vi "HiPace1200_Main.vi"() -> ()   [LabVIEW 2019]
panel:
  in  "audio_onoff":bool=TRUE caption="Audio\nAlarm"
  in  "control_onoff":bool=TRUE caption="Control"
  out "ack_ok":bool=TRUE
  out "motor_onoff":bool
  out "pump_st_onoff":bool
  out "temp_rotor":i16 caption="Rotor"
  out "temp_motor":i16 caption="Motor"
  out "temp_bearng":i16 caption="Bearing"
  out "temp_pmp_bot":i16 caption="Pump Bottom"
  out "temp_elec":i16 caption="Electric"
  out "temp_pwr_stg":i16 caption="Power Stage"
  out "gas_flow":i16 caption="sccm"
  out "accel":i16 caption="Accel."
  out "rot_speed_nom":i16 caption="Nominal"
  out "rot_speed_sp":i16 caption="Set Point"
  out "rot_speed_r":i16 caption="Reading"
  out "error_code":string caption="Error Code"
  in  "reconnect":bool
  in  "ack_error":bool
  in  "turn_off_motor":bool
  in  "turn_on_motor":bool
  in  "turn_off_pump_st":bool
  in  "turn_on_pump_st":bool
  in  "device_addr":u16=1 caption="Device addr."
  in  "port":u16=4196 caption="Port"
  in  "ip_addr":string="192.168.24.133" caption="IP addr."
  out "time":timestamp caption="Time" format="%<%Y-%m-%d %H:%M:%S>T"
  out "status":bool caption="Comm. status"
  in  "interval":u32=5000 caption="Interval"
  in  "stop":bool
  # "HiPace 1200:  Secondary IVC Pump"
  # "Pump Station"
  # "Rotation Speed"
  # "Hz"
  # "Hz"
  # "Hz"
  # "rpm/s"
  # "Temperature"
  # "Turbo Motor"
  # "degC"
  # "degC"
  # "degC"
  # "degC"
  # "degC"
  # "Error Code"
  # "degC"
  # "Gas Flow"
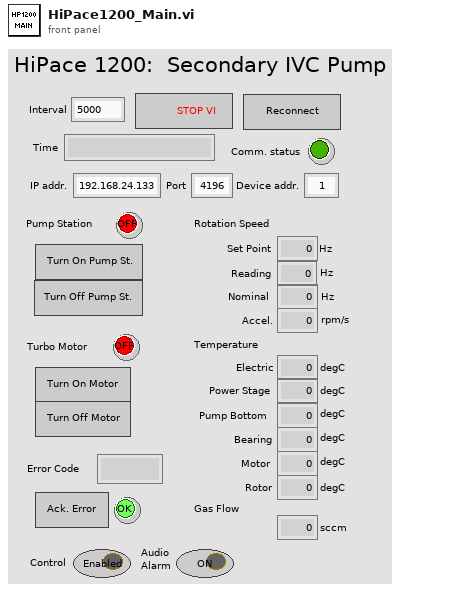
[diagram p1: front panel]
types:
  T1 = enum8{"Enabled", "Disabled", "Disabled and Grayed Out"}
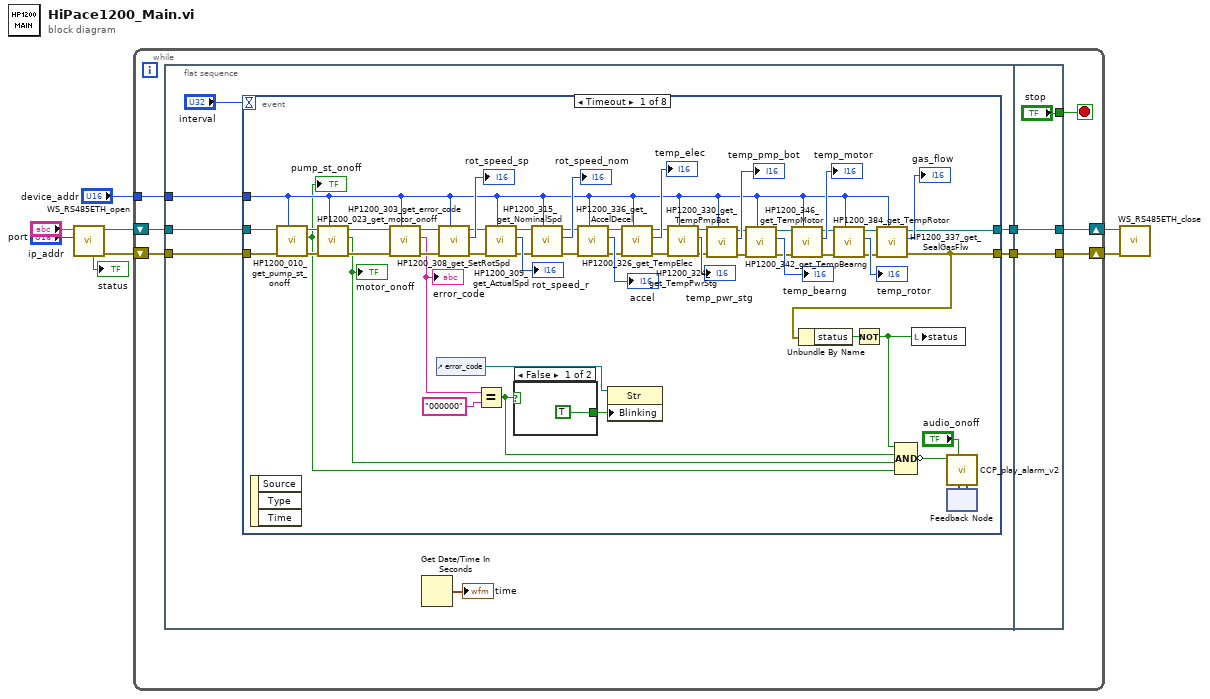
[diagram p0: block diagram]
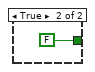
[diagram p2: hidden frame]
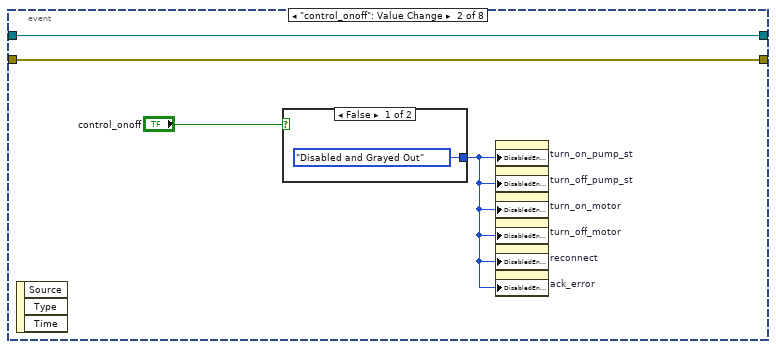
[diagram p3: hidden frame]
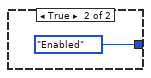
[diagram p4: hidden frame]
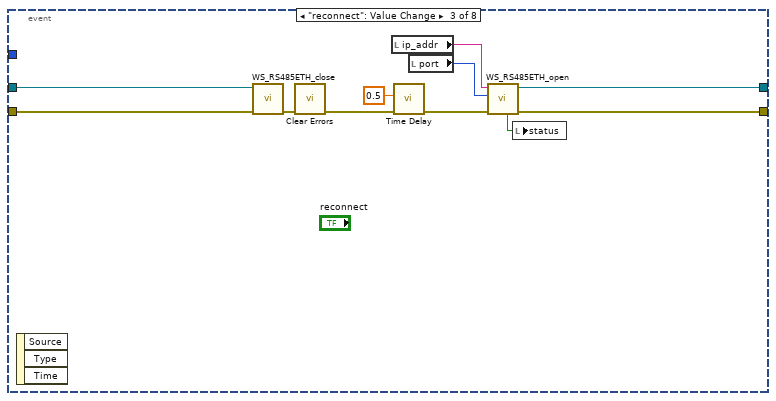
[diagram p5: hidden frame]
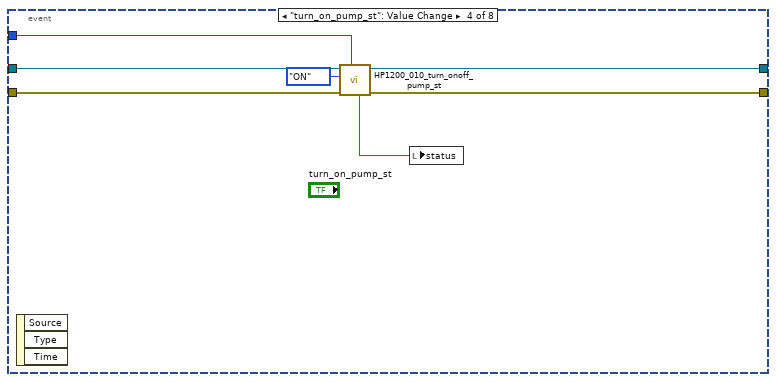
[diagram p6: hidden frame]
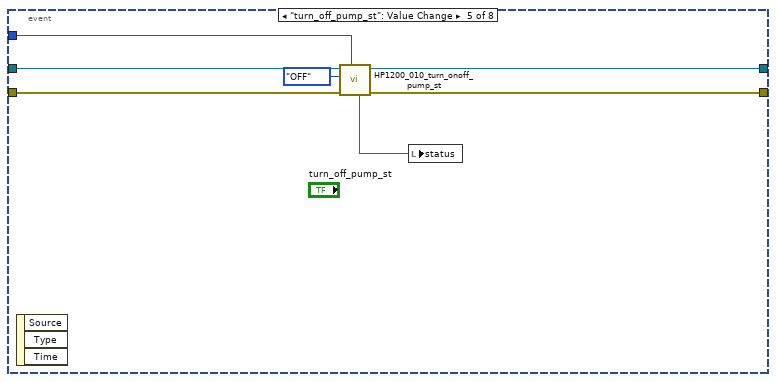
[diagram p7: hidden frame]
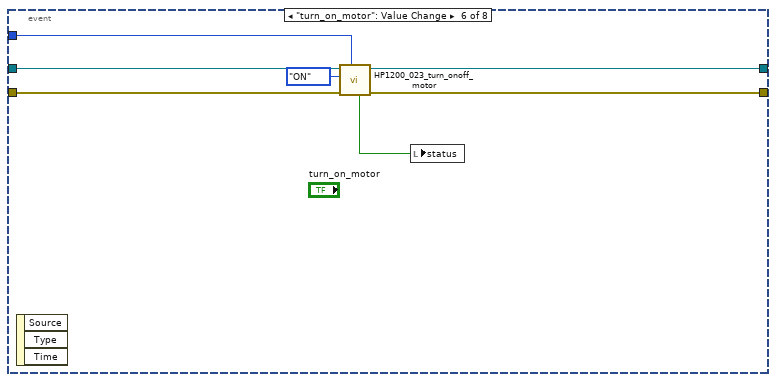
[diagram p8: hidden frame]
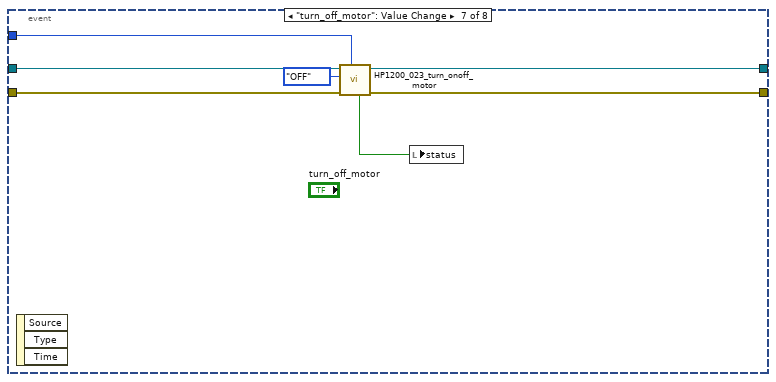
[diagram p9: hidden frame]
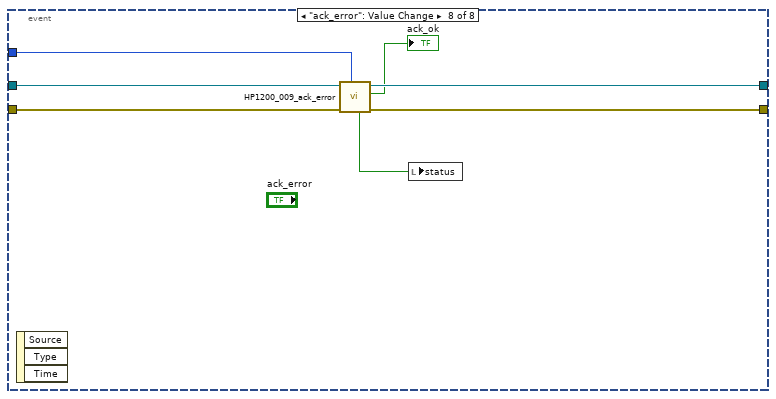
[diagram p10: hidden frame]
diagram:
  n1 = call "WS_RS485ETH_open.vi"("port"="port", "ip_addr"="ip_addr") -> ("error out"=w6:errorcluster, "conn_id"=w8:refnum<k5>, "status"=→"status":bool)  [unwired: 7 in]
  n2 = while {
    tunnel: "device_addr" -> [w9]
    shift-right: [w13] -> w7
    shift-left: w8 -> [w15]
    shift-right: [w10] -> w5
    shift-left: w6 -> [w12]
    stop <- w16 stop-if-true
    n3 = flat-sequence {
      tunnel: w15 -> [w23]
      tunnel: [w22] -> w14
      tunnel: w12 -> [w21]
      tunnel: [w20] -> w11
      tunnel: w9 -> [w18]
      tunnel: ["stop"] -> w16
      tunnel: w14 -> [w134]
      tunnel: [w134] -> w13
      tunnel: w11 -> [w133]
      tunnel: [w133] -> w10
      frame #0 {
        n4 = event shown="[0] Timeout" {
          selector: _ -> [_ _ _ _ _ _ _ _]
          dyn-events: _ -> [_ _ _ _ _ _ _ _]
          timeout: "interval" -> [_ _ _ _ _ _ _ _]
          tunnel: w23 -> [w40 w84 w97 w104 w111 w118 w125 w132]
          tunnel: [w45 w84 w95 w102 w109 w116 w123 w130] -> w22
          tunnel: w21 -> [w39 w83 w96 w103 w110 w117 w124 w131]
          tunnel: [w26 w83 w94 w101 w108 w115 w122 w129] -> w20
          tunnel: w18 -> [w34 _ _ w100 w107 w114 w121 w128]
          event Timeout {
            n5 = event-data() -> ()  [unwired: 1 in, 3 out]
            n6 = call "HP1200_010_get_pump_st_onoff.vi"("device_addr"=w34, "error in"=w39, "conn_id_in"=w40) -> ("error out"=w37:errorcluster, "onoff"=w31:bool, "conn_id_out"=w38:refnum<k5>)  [unwired: 3 in, 3 out]
            "pump_st_onoff" <- w31
            n7 = call "HP1200_023_get_motor_onoff.vi"("device_addr"=w34, "error in"=w37, "conn_id_in"=w38) -> ("error out"=w36:errorcluster, "motor_onoff"=w32:bool, "conn_id_out"=w35:refnum<k5>)  [unwired: 3 in, 3 out]
            "motor_onoff" <- w32
            n8 = call "HP1200_303_get_error_code.vi"("device_addr"=w34, "error in"=w36, "conn_id_in"=w35) -> ("error out"=w66:errorcluster, "error_code"=w41:string, "conn_id_out"=w67:refnum<k5>)  [unwired: 4 in, 2 out]
            "error_code" <- w41
            n9 = control-ref of="error_code"() -> (w43:refnum<vi>)
            n10 = call "HP1200_308_get_SetRotSpd.vi"("device_addr"=w34, "error in"=w66, "conn_id_in"=w67) -> ("error out"=w64:errorcluster, "rot_speed"=→"rot_speed_sp":i16, "conn_id_out"=w65:refnum<k5>)  [unwired: 4 in, 2 out]
            n11 = Equal?(x=w41, y="000000") -> (x = y?=w33:bool)
            n12 = call "HP1200_309_get_ActualSpd.vi"("device_addr"=w34, "error in"=w64, "conn_id_in"=w65) -> ("error out"=w62:errorcluster, "rot_speed"=→"rot_speed_r":i16, "conn_id_out"=w63:refnum<k5>)  [unwired: 4 in, 2 out]
            n13 = case shown="False" w33 {
              tunnel: [TRUE ("Blinking") FALSE ("Blinking")] -> w42
              frame False {
              }
              frame True {
              }
            }
            n14 = call "HP1200_315_get_NominalSpd.vi"("device_addr"=w34, "error in"=w62, "conn_id_in"=w63) -> ("error out"=w60:errorcluster, "rot_speed"=→"rot_speed_nom":i16, "conn_id_out"=w61:refnum<k5>)  [unwired: 4 in, 2 out]
            n15 = call "HP1200_336_get_AccelDecel.vi"("device_addr"=w34, "error in"=w60, "conn_id_in"=w61) -> ("error out"=w58:errorcluster, "acc"=→"accel":i16, "conn_id_out"=w59:refnum<k5>)  [unwired: 4 in, 2 out]
            n16 = property class="Str"(reference=w43, "Blinking"=w42) -> ()  [unwired: 1 in, 2 out]
            n17 = call "HP1200_326_get_TempElec.vi"("device_addr"=w34, "error in"=w58, "conn_id_in"=w59) -> ("error out"=w56:errorcluster, "temp"=→"temp_elec":i16, "conn_id_out"=w57:refnum<k5>)  [unwired: 4 in, 2 out]
            n18 = call "HP1200_324_get_TempPwrStg.vi"("device_addr"=w34, "error in"=w56, "conn_id_in"=w57) -> ("error out"=w54:errorcluster, "temp"=→"temp_pwr_stg":i16, "conn_id_out"=w55:refnum<k5>)  [unwired: 4 in, 2 out]
            n19 = call "HP1200_330_get_TempPmpBot.vi"("device_addr"=w34, "error in"=w54, "conn_id_in"=w55) -> ("error out"=w52:errorcluster, "temp"=→"temp_pmp_bot":i16, "conn_id_out"=w53:refnum<k5>)  [unwired: 4 in, 2 out]
            n20 = call "HP1200_342_get_TempBearng.vi"("device_addr"=w34, "error in"=w52, "conn_id_in"=w53) -> ("error out"=w48:errorcluster, "temp"=→"temp_bearng":i16, "conn_id_out"=w49:refnum<k5>)  [unwired: 4 in, 2 out]
            n21 = call "HP1200_346_get_TempMotor.vi"("device_addr"=w34, "error in"=w48, "conn_id_in"=w49) -> ("error out"=w50:errorcluster, "temp"=→"temp_motor":i16, "conn_id_out"=w51:refnum<k5>)  [unwired: 4 in, 2 out]
            n22 = call "HP1200_384_get_TempRotor.vi"("device_addr"=w34, "error in"=w50, "conn_id_in"=w51) -> ("error out"=w46:errorcluster, "temp"=→"temp_rotor":i16, "conn_id_out"=w47:refnum<k5>)  [unwired: 4 in, 2 out]
            n23 = call "HP1200_337_get_SealGasFlw.vi"("device_addr"=w34, "error in"=w46, "conn_id_in"=w47) -> ("error out"=w26:errorcluster, "flow"=→"gas_flow":i16, "conn_id_out"=w45:refnum<k5>)  [unwired: 4 in, 2 out]
            n24 = Unbundle By Name(w26) -> ("status"=w25:bool)
            n25 = Not(x=w25) -> (.not. x?=w24:bool)
            n26 = Compound Arithmetic op=AND(w24, w33, w32, w31) -> (invert w27:bool)
            n27 = local write "status"(w24) -> ()
            n28 = feedback #1() -> (w29:timestamp[])  [unwired: 1 in]
            n29 = call "CCP_play_alarm_v2.vi"("time_last_in"=w29, "audio_onoff"="audio_onoff", "error"=w27) -> ("time_last_out"=w30:timestamp[])  [unwired: 8 in]
            n30 = feedback-in #1(w30) -> ()
          }
          event "control_onoff": Value Change {
            n31 = event-data() -> ()  [unwired: 1 in, 3 out]
            n32 = case shown="False" "control_onoff" {
              tunnel: [T1."Disabled and Grayed Out" ("Disabled") T1."Enabled" ("Disabled")] -> w81
              frame False {
              }
              frame True {
              }
            }
            n33 = property on="turn_on_pump_st" class="Bool"("DisabledEnum"=w81) -> ()  [unwired: 2 in, 2 out]
            n34 = property on="turn_off_pump_st" class="Bool"("DisabledEnum"=w81) -> ()  [unwired: 2 in, 2 out]
            n35 = property on="turn_on_motor" class="Bool"("DisabledEnum"=w81) -> ()  [unwired: 2 in, 2 out]
            n36 = property on="turn_off_motor" class="Bool"("DisabledEnum"=w81) -> ()  [unwired: 2 in, 2 out]
            n37 = property on="reconnect" class="Bool"("DisabledEnum"=w81) -> ()  [unwired: 2 in, 2 out]
            n38 = property on="ack_error" class="Bool"("DisabledEnum"=w81) -> ()  [unwired: 2 in, 2 out]
          }
          event "reconnect": Value Change {
            n39 = event-data() -> ()  [unwired: 1 in, 3 out]
            n40 = call "WS_RS485ETH_close.vi"("error in"=w96, "conn_id"=w97) -> ("error out"=w91:errorcluster)  [unwired: 8 in, 1 out]
            n41 = call <vilib>:"Clear Errors.vi"("error in (no error)"=w91) -> ("error out"=w89:errorcluster)  [unwired: 5 in, 1 out]
            n42 = local read "ip_addr"() -> (w92:string)
            n43 = call "Time Delay"("error in (no error)"=w89, "Delay Time (s)"=0.5) -> ("error out"=w88:errorcluster)  [unwired: 9 in]
            n44 = local read "port"() -> (w93:u16)
            n45 = call "WS_RS485ETH_open.vi"("error in"=w88, "port"=w93, "ip_addr"=w92) -> ("error out"=w94:errorcluster, "conn_id"=w95:refnum<k5>, "status"=w90:bool)  [unwired: 6 in]
            n46 = local write "status"(w90) -> ()
          }
          event "turn_on_pump_st": Value Change {
            n47 = event-data() -> ()  [unwired: 1 in, 3 out]
            n48 = call "HP1200_010_turn_onoff_pump_st.vi"("device_addr"=w100, "error in"=w103, "onoff"=enum16{"ON", "OFF"}."ON", "conn_id_in"=w104) -> ("error out"=w101:errorcluster, "conn_id_out"=w102:refnum<k5>, "status"=w98:bool)  [unwired: 3 in, 2 out]
            n49 = local write "status"(w98) -> ()
          }
          event "turn_off_pump_st": Value Change {
            n50 = event-data() -> ()  [unwired: 1 in, 3 out]
            n51 = call "HP1200_010_turn_onoff_pump_st.vi"("device_addr"=w107, "error in"=w110, "onoff"=enum16{"ON", "OFF"}."OFF", "conn_id_in"=w111) -> ("error out"=w108:errorcluster, "conn_id_out"=w109:refnum<k5>, "status"=w105:bool)  [unwired: 3 in, 2 out]
            n52 = local write "status"(w105) -> ()
          }
          event "turn_on_motor": Value Change {
            n53 = event-data() -> ()  [unwired: 1 in, 3 out]
            n54 = call "HP1200_023_turn_onoff_motor.vi"("device_addr"=w114, "error in"=w117, "onoff"=enum16{"ON", "OFF"}."ON", "conn_id_in"=w118) -> ("error out"=w115:errorcluster, "conn_id_out"=w116:refnum<k5>, "status"=w112:bool)  [unwired: 3 in, 2 out]
            n55 = local write "status"(w112) -> ()
          }
          event "turn_off_motor": Value Change {
            n56 = event-data() -> ()  [unwired: 1 in, 3 out]
            n57 = call "HP1200_023_turn_onoff_motor.vi"("device_addr"=w121, "error in"=w124, "onoff"=enum16{"ON", "OFF"}."OFF", "conn_id_in"=w125) -> ("error out"=w122:errorcluster, "conn_id_out"=w123:refnum<k5>, "status"=w119:bool)  [unwired: 3 in, 2 out]
            n58 = local write "status"(w119) -> ()
          }
          event "ack_error": Value Change {
            n59 = event-data() -> ()  [unwired: 1 in, 3 out]
            n60 = call "HP1200_009_ack_error.vi"("device_addr"=w128, "error in"=w131, "conn_id_in"=w132) -> ("error out"=w129:errorcluster, "ack_ok"=→"ack_ok":bool, "conn_id_out"=w130:refnum<k5>, "status"=w127:bool)  [unwired: 3 in, 2 out]
            n61 = local write "status"(w127) -> ()
          }
        }
        n62 = Get Date/Time In Seconds() -> (seconds since 1Jan1904=→"time":timestamp)
      }
      frame #1 {
      }
    }
  }
  n63 = call "WS_RS485ETH_close.vi"("error in"=w5, "conn_id"=w7) -> ()  [unwired: 8 in, 2 out]
